vi "fftw_destroy_plan.vi"(8 "error in (no error)":errorcluster, 11 "*plan":u64) -> (0 "error out":errorcluster)   [LabVIEW 2020, in "FFTWDLL.lvlib"]
doc: "Destroy FFTW plan."
uses:
  FFTWDLL.lvlib
  dll/libfftw3-3.dll
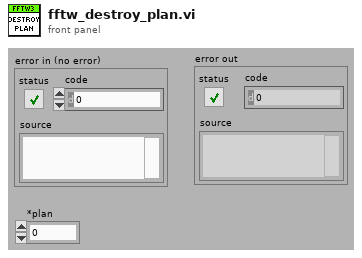
[diagram p1: front panel]
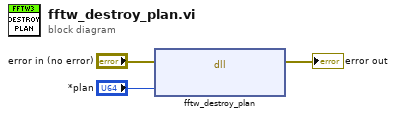
[diagram p0: block diagram]
diagram:
  n1 = dll-call lib="E:/LV_prog/maslan/fftw3-dll-labview/dll/libfftw3-3.dll" fn="fftw_destroy_plan"(error in="error in (no error)", "*plan"="*plan") -> (error out=→"error out":errorcluster)  [unwired: 4 in, 1 out]
